vi "Read Data.vi"(8 "error in (no error)":errorcluster, 10 "Count":i32, 11 "Stream in":refnum<class "Stream.lvclass">) -> (0 "error out":errorcluster, 2 "Data":string, 3 "Stream out":refnum<class "Stream.lvclass">)   [LabVIEW 2020, in "IO.lvlib" / "Stream.lvclass"]
uses:
  Stream.lvclass
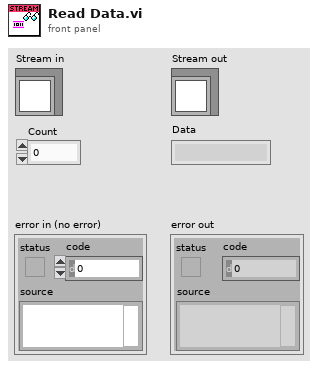
[diagram p1: front panel]
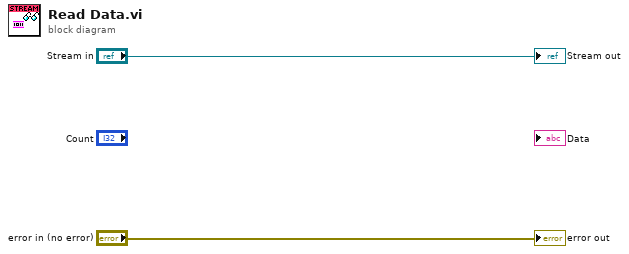
[diagram p0: block diagram]
diagram:
  "error out" <- "error in (no error)"
  "Stream out" <- "Stream in"
